vi "Auto Hopper and Gear.vi"(9 "openGear":dbl, 10 "Fill Hopper?":dbl) -> ()   [LabVIEW 2016]
uses:
  Common Code/Intake Modes.ctl
  Robot Global Data.vi
panel:
  out "yea":bool
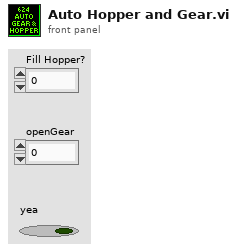
[diagram p1: front panel]
types:
  T1 = typedef "Intake Modes.ctl" = enum16{"Manual", "Auto"}
  T2 = typedef "Intake Control Cluster.ctl" = cluster{"Intake Mode":T1, "Intake Auto Command":T3, "Intake Current Trip State":T4, "Engage traction for gear load?":bool, "Wings open?":bool, "Manual Angle Power":dbl, "Manual Roller Power":dbl}
  T3 = typedef "Intake Auto States.ctl" = enum16{"Zero", "Unload", "Load", "Idle ", "FeederStation"}
  T4 = typedef "Intake Trip States.ctl" = enum16{"Normal", "Backward Tripped", "Forward Tripped"}
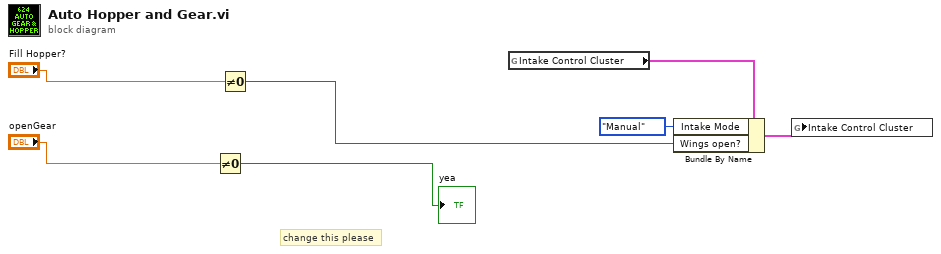
[diagram p0: block diagram]
diagram:
  # "change this please"
  n1 = Not Equal To 0?(x="openGear") -> (x != 0?=→"yea":bool)
  n2 = Not Equal To 0?(x="Fill Hopper?") -> (x != 0?=w3:bool)
  n3 = global read "Robot Global Data.vi" "Intake Control Cluster"() -> (w7:T2)
  n4 = Bundle By Name(cluster=w7, "Intake Mode"=Intake_Modes."Manual", "Wings open?"=w3) -> (w6:T2)
  n5 = global write "Robot Global Data.vi" "Intake Control Cluster"(w6) -> ()
